vi "IDrawable Draw.vi"(7 "Drawing Settings":T1, 8 "error in (no error)":errorcluster, 10 "2D Picture":picture, 11 "IDrawable in":refnum<class "IDrawable.lvclass">) -> (0 "error out":errorcluster, 2 "2D Picture out":picture, 3 "IDrawable out":refnum<class "IDrawable.lvclass">)   [LabVIEW 2020, in "IDrawable.lvclass"]
uses:
  IDrawable.lvclass
  Drawing Settings STYP.ctl
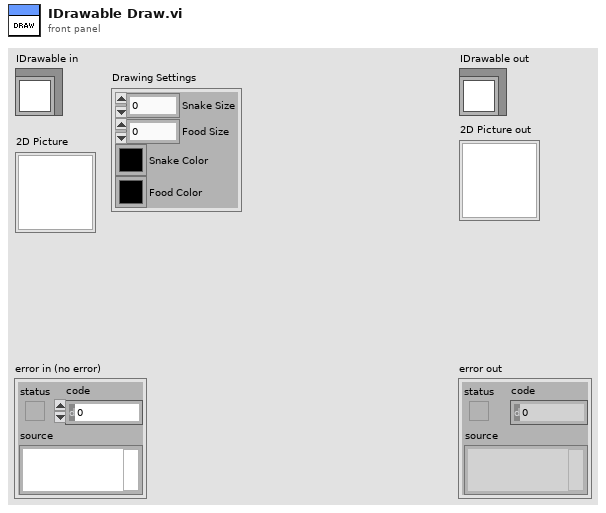
[diagram p1: front panel]
types:
  T1 = typedef "Drawing Settings STYP.ctl" = cluster{"Snake Size":u32, "Food Size":u32, "Snake Color":u32, "Food Color":u32}
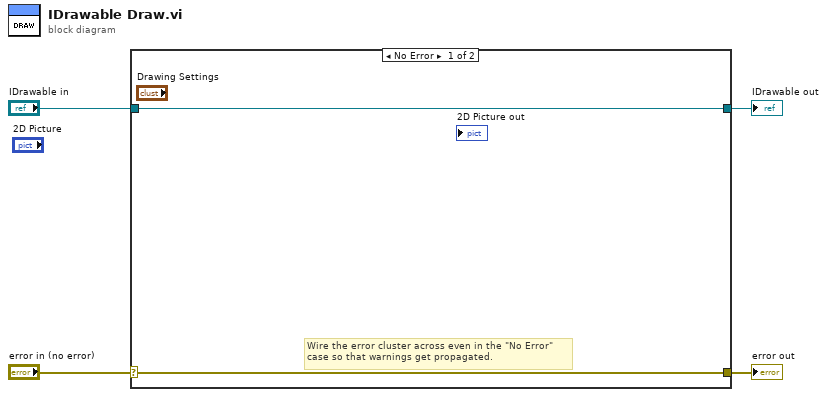
[diagram p0: block diagram]
diagram:
  n1 = case shown="No Error" "error in (no error)" {
    selector: "error in (no error)" -> [w5 w8]
    tunnel: [w5 w8] -> w3
    tunnel: [w6 w7] -> w1
    tunnel: "IDrawable in" -> [w6 w7]
    frame No Error {
      # "Wire the error cluster across even in the \"No Error\"\ncase so that warnings get propagated."
    }
    frame Error {
    }
  }
  "error out" <- w3
  "IDrawable out" <- w1
